vi "Actor Core.vi"(8 "error in":errorcluster, 11 "CS++DSCMonitor in":refnum<class "CS++DSCMonitor.lvclass">) -> (0 "error out":errorcluster, 3 "Actor out":refnum<class "Actor.lvclass">)   [LabVIEW 2014, in "CS++DSCMonitor.lvlib" / "CS++DSCMonitor.lvclass"]
doc: "(<B>Filename</B>: Actor Framework.lvlib:Actor.lvclass:Actor Core.vi)\n\nReceives messages to the actor, reacts to them, and initiates any error handling that may shut the actor down.\n\nDescendant classes may override this VI to append parallel tasks for the actor to complete while it handles messages. Overrides use the Call Parent Method node."
uses:
  CS++DSCMonitor.lvclass
  CSPP_Core/Actors/CS++SVMonitor/CS++SVMonitor.lvclass
  CSPP_Core/Actors/CS++BaseActor/CS++BaseActor.lvclass
  <vilib>/lvdsc/NI_DSC.lvlib
  <vilib>/ActorFramework/Actor/Actor.lvclass
  CSPP_Core/Actors/CS++PVMonitor Messages/CS++PVUpdate Msg/CS++PVUpdate Msg.lvclass
  CSPP_Core/Actors/CS++PVMonitor Messages/CS++AEUpdate Msg/CS++AEUpdate Msg.lvclass
  CSPP_Core/Classes/CS++ProcessVariables/AlarmEvent/AE.lvclass
  CSPP_Core/Classes/CS++ProcessVariables/AE Type.ctl
  CSPP_Core/Classes/CS++ProcessVariables/CS++ProcessVariables.lvlib
  CSPP_Core/Classes/CS++ProcessVariables/ProcessVariable/PV.lvclass
  <vilib>/ActorFramework/Report Error Msg/Report Error Msg.lvclass
  <vilib>/ActorFramework/Message Enqueuer/Message Priority.ctl
  <vilib>/ActorFramework/Message Enqueuer/Message Enqueuer.lvclass
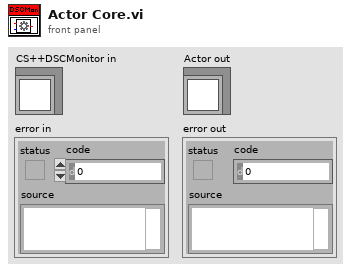
[diagram p1: front panel]
types:
  T1 = typedef "Actor Framework.lvlib/Message Enqueuer.lvclass/Message Priority.ctl" = enum16{"Low", "Normal", "High"}
  T2 = typedef "CS++ProcessVariables.lvlib/AE Type.ctl" = enum16{"Event", "HI_HI", "HI", "LO", "LO_LO", "Boolean", "ROC", "Invalid", "Other"}
  T3 = cluster{"Stop":refnum<user-event>, "PV Connections":refnum<user-event>}
  T4 = cluster{"PV URL":string, "Observers":cluster{"Enqueuer":refnum<class "Message Enqueuer.lvclass">, "CS++PVUpdate Msg":refnum<class "CS++PVUpdate Msg.lvclass">}[]}[]
  T5 = cluster{"AE URL":string, "Observers":cluster{"Enqueuer":refnum<class "Message Enqueuer.lvclass">, "CS++AEUpdate Msg":refnum<class "CS++AEUpdate Msg.lvclass">}[]}[]
  T6 = cluster{"PV URL":string, "Observers":cluster{"Enqueuer":refnum<class "Message Enqueuer.lvclass">, "CS++PVUpdate Msg":refnum<class "CS++PVUpdate Msg.lvclass">}[]}
  T7 = cluster{"Enqueuer":refnum<class "Message Enqueuer.lvclass">, "CS++PVUpdate Msg":refnum<class "CS++PVUpdate Msg.lvclass">}[]
  T8 = cluster{"AE URL":string, "Observers":cluster{"Enqueuer":refnum<class "Message Enqueuer.lvclass">, "CS++AEUpdate Msg":refnum<class "CS++AEUpdate Msg.lvclass">}[]}
  T9 = cluster{"Enqueuer":refnum<class "Message Enqueuer.lvclass">, "CS++AEUpdate Msg":refnum<class "CS++AEUpdate Msg.lvclass">}[]
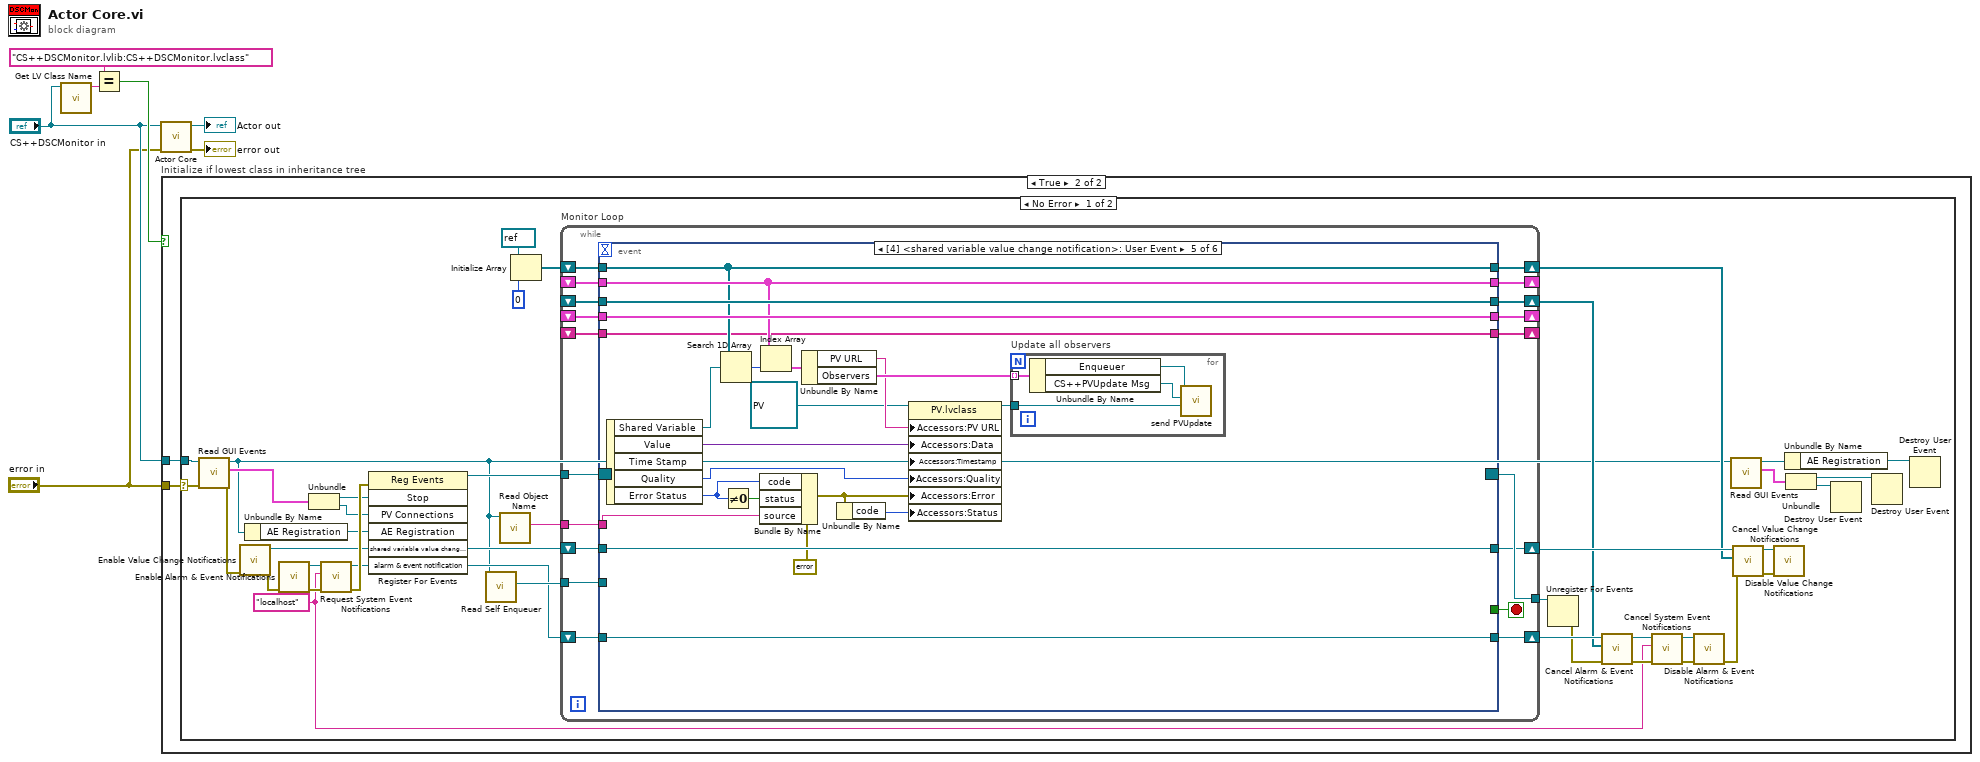
[diagram p0: block diagram]
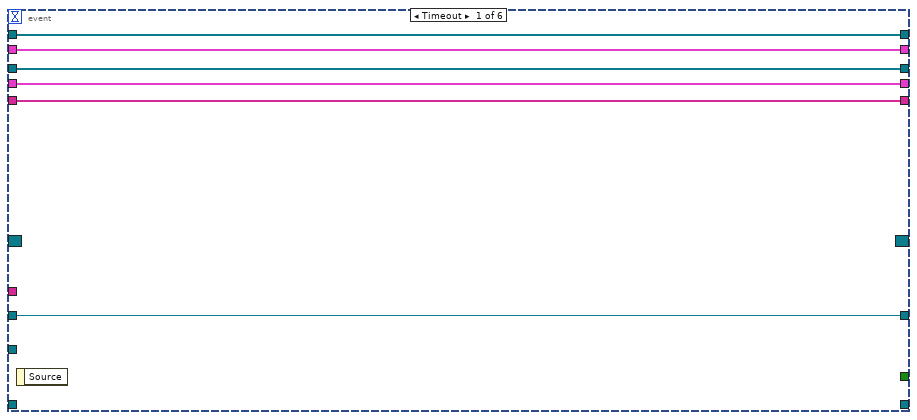
[diagram p3: hidden frame]
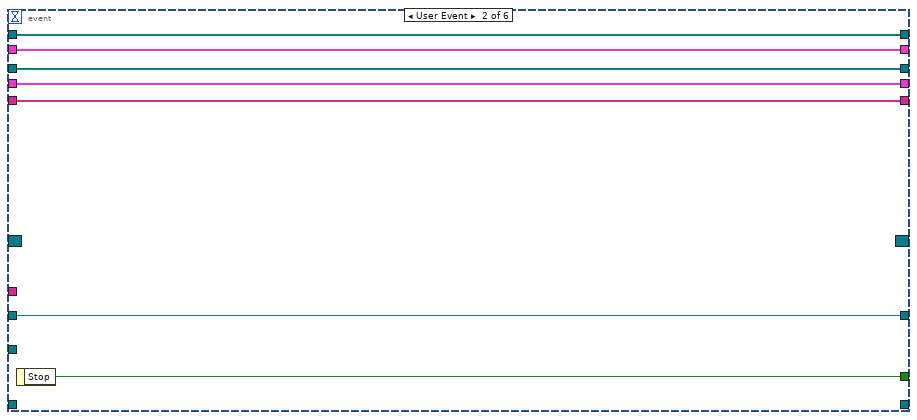
[diagram p4: hidden frame]
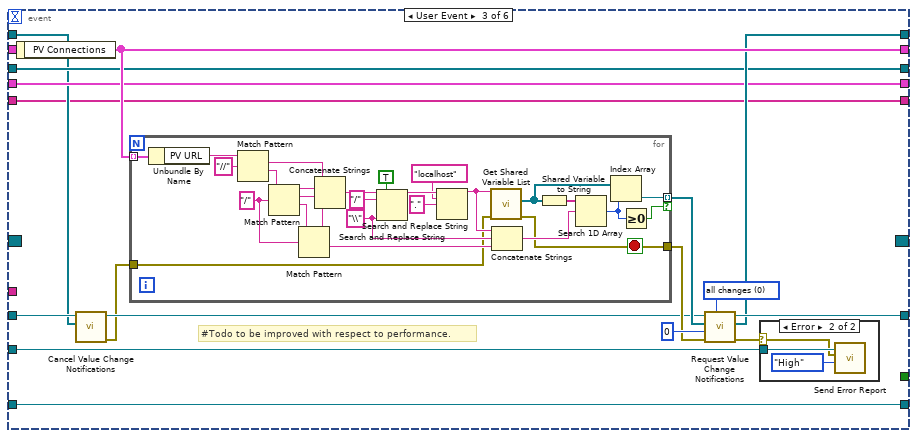
[diagram p5: hidden frame]
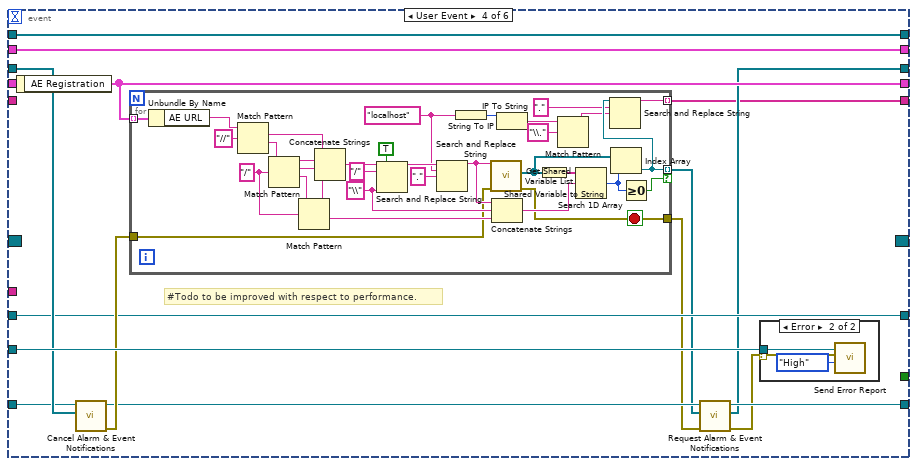
[diagram p7: hidden frame]
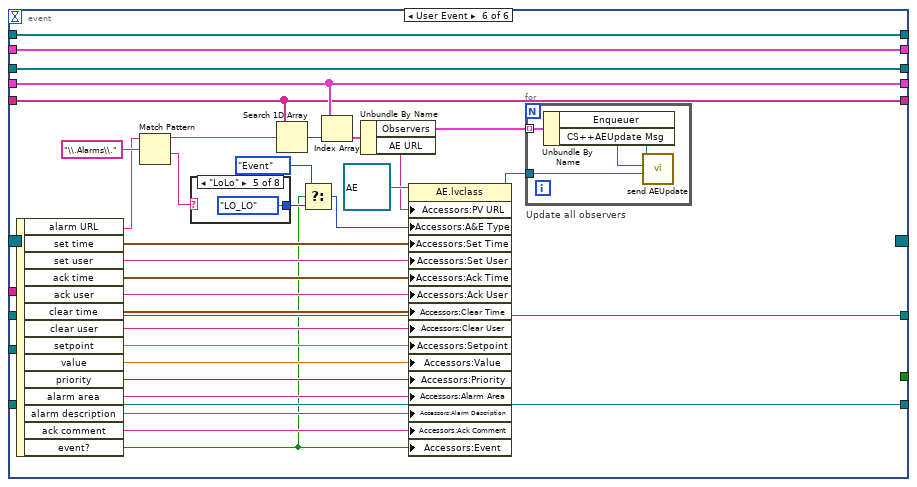
[diagram p9: hidden frame]
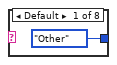
[diagram p10: hidden frame]
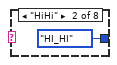
[diagram p11: hidden frame]
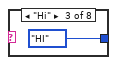
[diagram p12: hidden frame]
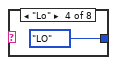
[diagram p13: hidden frame]
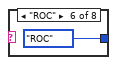
[diagram p14: hidden frame]
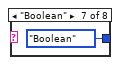
[diagram p15: hidden frame]
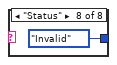
[diagram p16: hidden frame]
diagram:
  n1 = call <vilib>:"Get LV Class Name.vi"("object"="CS++DSCMonitor in") -> ("class name"=w6:string)  [unwired: 9 in, 1 out]
  n2 = Equal?(x="CS++DSCMonitor.lvlib:CS++DSCMonitor.lvclass" ("class name"), y=w6) -> (x = y?=w3:bool)
  n3 = call-parent "Actor Core.vi"("error in"="error in", "CS++SVMonitor in"="CS++DSCMonitor in") -> ("error out"=→"error out":errorcluster, "Actor out"=→"Actor out":refnum<class "Actor.lvclass">)  [unwired: 8 in]
  n4 = case "Initialize if lowest class in inheritance tree" shown="True" w3 {
    tunnel: "error in" -> [_ w9]
    tunnel: "CS++DSCMonitor in" -> [_ w8]
    frame False {
    }
    frame True {
      n5 = case shown="No Error" w9 {
        selector: w9 -> [w20 _]
        tunnel: w8 -> [w19 _]
        frame No Error {
          w18 = "localhost" ("server (localhost)")
          n6 = call "Read GUI Events.vi"("error in (no error)"=w20, "CS++SVMonitor in"=w19) -> ("error out"=w25:errorcluster, "GUI Events"=w24:T3, "CS++SVMonitor out"=w13:refnum<class "CS++DSCMonitor.lvclass">)  [unwired: 7 in]
          n7 = call <vilib>:"Enable Value Change Notifications.vi"("error in (no error)"=w25) -> ("error out"=w26:errorcluster, "shared variable value change notification"=w17:refnum<user-event>)  [unwired: 9 out]
          n8 = Unbundle By Name(w13) -> ("AE Registration"=w27:refnum<user-event>)
          n9 = call <vilib>:"Enable Alarm & Event Notifications.vi"("error in (no error)"=w26) -> ("error out"=w29:errorcluster, "alarm & event notification"=w28:refnum<user-event>)  [unwired: 9 out]
          n10 = Unbundle(w24) -> ("Stop"=w23:refnum<user-event>, "PV Connections"=w22:refnum<user-event>)
          n11 = call <vilib>:"Request System Event Notifications.vi"("error in (no error)"=w29, "server (localhost)"=w18, "notification refnum"=w28) -> ("error out"=w30:errorcluster, "alarm & event notification"=w16:refnum<user-event>)  [unwired: 6 in, 1 out]
          n12 = register-events(error in=w30, w23, w22, w27, w17, w16) -> (reference out=w21:refnum<event-registration>)  [unwired: 1 in, 1 out]
          n13 = call <vilib>:"Read Self Enqueuer.vi"("Actor"=w13) -> ("Self Enqueuer"=w44:refnum<class "Message Enqueuer.lvclass">)  [unwired: 10 in]
          n14 = call "Read Object Name.vi"("CS++BaseActor in"=w13) -> ("Object Name"=w46:string)  [unwired: 8 in, 2 out]
          n15 = Initialize Array(refnum<k21> refnum ("Shared Variable"), 0 ("dimension size")) -> (w43:refnum<k21>[])
          n16 = while "Monitor Loop" {
            tunnel: w21 -> [w67]
            tunnel: [w65] -> w48
            shift-right: [w63] -> w40
            shift-left: w43 -> [w64]
            shift-right: [w62] -> _
            shift-left: _ -> [w61]
            shift-right: [w59] -> w42
            shift-left: w17 -> [w60]
            tunnel: w46 -> [w58]
            tunnel: w44 -> [w57]
            shift-right: [w56] -> w38
            shift-left: w16 -> [w55]
            shift-right: [w52] -> w35
            shift-left: _ -> [w54]
            shift-right: [w53] -> _
            shift-left: _ -> [w51]
            shift-right: [w50] -> _
            shift-left: _ -> [w49]
            stop <- w66 stop-if-true
            n17 = event shown="[4] <shared variable value change notification>: User Event" {
              selector: w67 -> [_ _ _ _ _ _]
              dyn-events: [_ _ _ _ _ _] -> w65
              timeout: _ -> [_ _ _ _ _ _]
              tunnel: [_ w80 _ _ _ _] -> w66
              tunnel: w64 -> [w73 w79 w82 w138 w193 w235]
              tunnel: [w73 w79 w89 w138 w193 w235] -> w63
              tunnel: [w72 w78 w96 w141 w194 w237] -> w62
              tunnel: w61 -> [w72 w78 _ w141 w194 w237]
              tunnel: w60 -> [w71 w77 w85 w135 w201 w238]
              tunnel: [w71 w77 w97 w135 w201 w238] -> w59
              tunnel: w58 -> [_ _ _ _ w191 _]
              tunnel: w57 -> [_ _ w91 w142 _ _]
              tunnel: [_ _ w90 w133 w197 w236] -> w56
              tunnel: w55 -> [_ _ w90 w136 w197 w236]
              tunnel: w54 -> [w69 w76 w87 w139 w196 w234]
              tunnel: [w70 w75 w86 w140 w195 w233] -> w53
              tunnel: [w69 w76 w87 w130 w196 w234] -> w52
              tunnel: w51 -> [w70 w75 w86 _ w195 w233]
              tunnel: [w68 w74 w81 w128 w188 w229] -> w50
              tunnel: w49 -> [w68 w74 w81 _ w188 w229]
              event Timeout {
                n18 = event-data() -> ()  [unwired: 1 in, 1 out]
              }
              event User Event {
                n19 = event-data() -> ("Stop"=w80:bool)  [unwired: 1 in]
              }
              event User Event {
                w95 = u16 0 items=["all changes", "value changes only"] ("request changes (all changes)")
                # "#Todo to be improved with respect to performance."
                n20 = event-data() -> ("PV Connections"=w96:T4)  [unwired: 1 in]
                n21 = call <vilib>:"Cancel Value Change Notifications.vi"("shared variables"=w82, "notification refnum"=w85) -> ("error out"=w83:errorcluster, "shared variable value change notification"=w84:refnum<user-event>)  [unwired: 1 in, 7 out]
                n22 = for {
                  tunnel: w96 -> [w127] mode=indexing
                  tunnel: [w115] -> w88 mode=indexing if=w114
                  tunnel: [w102] -> w93
                  tunnel: w83 -> [w101]
                  stop <- w102 stop-if-true
                  w103 = "\\" ("replace string (\"\")")
                  w123 = "/" ("regular expression")
                  n23 = Unbundle By Name(w127) -> ("PV URL"=w117:string)
                  n24 = Match Pattern(string=w117, regular expression="//") -> (match substring=w122:string, after substring=w125:string)  [unwired: 1 in, 2 out]
                  n25 = Match Pattern(string=w125, regular expression=w123) -> (before substring=w121:string, match substring=w120:string, after substring=w124:string)  [unwired: 1 in, 1 out]
                  n26 = Match Pattern(string=w124, regular expression=w123) -> (before substring=w119:string, after substring=w109:string)  [unwired: 1 in, 2 out]
                  n27 = Concatenate Strings(w122, w121, w120, w119) -> (w112:string)
                  n28 = Search and Replace String(replace all?=TRUE ("replace all? (F)"), input string=w112, search string="/", replace string=w103) -> (result string=w107:string)  [unwired: 4 in, 3 out]
                  n29 = Search and Replace String(input string=w107, search string="localhost", replace string="." ("replace string (\"\")")) -> (result string=w104:string)  [unwired: 5 in, 3 out]
                  n30 = call <vilib>:"Get Shared Variable List.vi"("error in (no error)"=w101, "process name"=w104) -> ("error out"=w102:errorcluster, "shared variables"=w116:refnum<k21>[])  [unwired: 8 out]
                  n31 = Concatenate Strings(w104, w103, w109) -> (w108:string)
                  n32 = Shared Variable to String(1:w116) -> (0:w118:string[])
                  n33 = Search 1D Array(1D array=w118, element=w108) -> (index of element=w113:i32)  [unwired: 1 in]
                  n34 = Index Array(array=w116, index=w113) -> (element=w115:refnum<k21>)
                  n35 = Greater Or Equal To 0?(x=w113) -> (x >= 0?=w114:bool)
                }
                n36 = call <vilib>:"Request Value Change Notifications.vi"("request changes (all changes)"=w95, "error in (no error)"=w93, "updates to buffer (no buffer)"=u32 0, "shared variables"=w88, "notification refnum"=w84) -> ("error out"=w92:errorcluster, "shared variables out"=w89:refnum<k21>[], "shared variable value change notification"=w97:refnum<user-event>)  [unwired: 4 out]
                n37 = case shown="Error" w92 {
                  selector: w92 -> [_ w99]
                  tunnel: w91 -> [_ w100]
                  frame No Error {
                  }
                  frame Error {
                    n38 = call <vilib>:"Send Error Report.vi"("Message Priority (Normal)"=Message_Priority."High", "Error From Sender"=w99, "Message Enqueuer"=w100) -> ()  [unwired: 8 in, 1 out]
                  }
                }
              }
              event User Event {
                # "#Todo to be improved with respect to performance."
                n39 = event-data() -> ("AE Registration"=w140:T5)  [unwired: 1 in]
                n40 = call <vilib>:"Cancel Alarm & Event Notifications.vi"("shared variables"=w139, "notification refnum"=w136) -> ("error out"=w137:errorcluster, "alarm & event notification"=w134:refnum<user-event>)  [unwired: 7 in, 1 out]
                n41 = for {
                  tunnel: w140 -> [w178] mode=indexing
                  tunnel: [w150] -> w129 mode=indexing if=w167
                  tunnel: [w157] -> w132
                  tunnel: w137 -> [w156]
                  tunnel: [w151] -> w128 mode=indexing
                  stop <- w157 stop-if-true
                  w153 = "localhost" ("search string")
                  w158 = "\\" ("replace string (\"\")")
                  w174 = "/" ("regular expression")
                  n42 = Unbundle By Name(w178) -> ("AE URL"=w152:string)
                  n43 = Match Pattern(string=w152, regular expression="//") -> (match substring=w173:string, after substring=w176:string)  [unwired: 1 in, 2 out]
                  n44 = Match Pattern(string=w176, regular expression=w174) -> (before substring=w172:string, match substring=w171:string, after substring=w175:string)  [unwired: 1 in, 1 out]
                  n45 = Match Pattern(string=w175, regular expression=w174) -> (before substring=w170:string, after substring=w162:string)  [unwired: 1 in, 2 out]
                  n46 = Concatenate Strings(w173, w172, w171, w170) -> (w165:string)
                  n47 = Search and Replace String(replace all?=TRUE ("replace all? (F)"), input string=w165, search string="/", replace string=w158) -> (result string=w160:string)  [unwired: 4 in, 3 out]
                  n48 = Search and Replace String(input string=w160, search string=w153, replace string="." ("replace string (\"\")")) -> (result string=w159:string)  [unwired: 5 in, 3 out]
                  n49 = String To IP(1:w153) -> (0:w155:u32)
                  n50 = call <vilib>:"Get Shared Variable List.vi"("error in (no error)"=w156, "process name"=w159) -> ("error out"=w157:errorcluster, "shared variables"=w168:refnum<k21>[])  [unwired: 8 out]
                  n51 = Concatenate Strings(w159, w158, w162) -> (w161:string)
                  n52 = IP To String(2:w155) -> (0:w154:string)  [unwired: 1 in]
                  n53 = Shared Variable to String(1:w168) -> (0:w169:string[])
                  n54 = Match Pattern(string=w154, regular expression="\\.") -> (before substring=w149:string)  [unwired: 1 in, 3 out]
                  n55 = Search 1D Array(1D array=w169, element=w161) -> (index of element=w166:i32)  [unwired: 1 in]
                  n56 = Index Array(array=w168, index=w166) -> (element=w150:refnum<k21>)
                  n57 = Search and Replace String(input string=w150, search string=".", replace string=w149) -> (result string=w151:string)  [unwired: 5 in, 3 out]
                  n58 = Greater Or Equal To 0?(x=w166) -> (x >= 0?=w167:bool)
                }
                n59 = call <vilib>:"Request Alarm & Event Notifications.vi"("error in (no error)"=w132, "shared variables"=w129, "notification refnum"=w134) -> ("error out"=w131:errorcluster, "shared variables out"=w130:refnum<k21>[], "alarm & event notification"=w133:refnum<user-event>)  [unwired: 6 out]
                n60 = case shown="Error" w131 {
                  selector: w131 -> [_ w144]
                  tunnel: w142 -> [_ w145]
                  frame No Error {
                  }
                  frame Error {
                    n61 = call <vilib>:"Send Error Report.vi"("Message Priority (Normal)"=Message_Priority."High", "Error From Sender"=w144, "Message Enqueuer"=w145) -> ()  [unwired: 8 in, 1 out]
                  }
                }
              }
              event User Event {
                n62 = event-data() -> ("Shared Variable"=w198:refnum<k21>, "Value"=w184:variant, "Time Stamp"=w183:timestamp, "Quality"=w181:u64, "Error Status"=w189:i32)  [unwired: 1 in]
                n63 = Search 1D Array(1D array=w193, element=w198) -> (index of element=w200:i32)  [unwired: 1 in]
                n64 = Not Equal To 0?(x=w189) -> (x != 0?=w190:bool)
                n65 = Bundle By Name(cluster=errorcluster {"status"=FALSE, "code"=0, "source"=""} ("Error"), "code"=w189, "status"=w190, "source"=w191) -> (w182:errorcluster)
                n66 = Index Array(array=w194, index=w200) -> (element=w199:T6)
                n67 = Unbundle By Name(w199) -> ("PV URL"=w185:string, "Observers"=w187:T7)
                n68 = Unbundle By Name(w182) -> ("code"=w186:i32)
                n69 = property class="PV.lvclass"(reference=refnum<class "PV.lvclass"> refnum ("PV"), "Accessors:PV URL"=w185, "Accessors:Data"=w184, "Accessors:Timestamp"=w183, "Accessors:Quality"=w181, "Accessors:Error"=w182, "Accessors:Status"=w186) -> (reference out=w180:refnum<class "PV.lvclass">)  [unwired: 1 in, 1 out]
                n70 = for "Update all observers" {
                  tunnel: w187 -> [w205] mode=indexing
                  tunnel: w180 -> [w202]
                  n71 = Unbundle By Name(w205) -> ("Enqueuer"=w204:refnum<class "Message Enqueuer.lvclass">, "CS++PVUpdate Msg"=w203:refnum<class "CS++PVUpdate Msg.lvclass">)
                  n72 = call "send PVUpdate.vi"("PV"=w202, "CS++PVUpdate Msg in"=w203, "Message Enqueuer in"=w204) -> ()  [unwired: 7 in, 2 out]
                }
              }
              event User Event {
                n73 = event-data() -> ("alarm URL"=w227:string, "set time"=w219:timestamp, "set user"=w218:string, "ack time"=w217:timestamp, "ack user"=w216:string, "clear time"=w215:timestamp, "clear user"=w214:string, "setpoint"=w213:dbl, "value"=w212:dbl, "priority"=w211:u32, "alarm area"=w210:string, "alarm description"=w209:string, "ack comment"=w208:string, "event?"=w207:bool)  [unwired: 1 in]
                n74 = Match Pattern(string=w227, regular expression="\\.Alarms\\.") -> (before substring=w225:string, after substring=w224:string)  [unwired: 1 in, 2 out]
                n75 = case shown="\"LoLo\"" w224 {
                  tunnel: [AE_Type."Other" ("A&E Type") AE_Type."HI_HI" ("A&E Type") AE_Type."HI" ("A&E Type") AE_Type."LO" ("A&E Type") AE_Type."LO_LO" ("A&E Type") AE_Type."ROC" ("A&E Type") AE_Type."Boolean" ("A&E Type") AE_Type."Invalid" ("A&E Type")] -> w221
                  frame Default {
                  }
                  frame "HiHi" {
                  }
                  frame "Hi" {
                  }
                  frame "Lo" {
                  }
                  frame "LoLo" {
                  }
                  frame "ROC" {
                  }
                  frame "Boolean" {
                  }
                  frame "Status" {
                  }
                }
                n76 = Search 1D Array(1D array=w229, element=w225) -> (index of element=w231:i32)  [unwired: 1 in]
                n77 = Select(t=AE_Type."Event" ("A&E Type"), s=w207, f=w221) -> (s? t:f=w222:T2)
                n78 = Index Array(array=w233, index=w231) -> (element=w230:T8)
                n79 = Unbundle By Name(w230) -> ("Observers"=w232:T9, "AE URL"=w220:string)
                n80 = property class="AE.lvclass"(reference=refnum<class "AE.lvclass"> refnum ("CS++ProcessVariables.lvlib:AE.lvclass"), "Accessors:PV URL"=w220, "Accessors:A&E Type"=w222, "Accessors:Set Time"=w219, "Accessors:Set User"=w218, "Accessors:Ack Time"=w217, "Accessors:Ack User"=w216, "Accessors:Clear Time"=w215, "Accessors:Clear User"=w214, "Accessors:Setpoint"=w213, "Accessors:Value"=w212, "Accessors:Priority"=w211, "Accessors:Alarm Area"=w210, "Accessors:Alarm Description"=w209, "Accessors:Ack Comment"=w208, "Accessors:Event"=w207) -> (reference out=w206:refnum<class "AE.lvclass">)  [unwired: 1 in, 1 out]
                n81 = for "Update all observers" {
                  tunnel: w232 -> [w250] mode=indexing
                  tunnel: w206 -> [w247]
                  n82 = Unbundle By Name(w250) -> ("Enqueuer"=w249:refnum<class "Message Enqueuer.lvclass">, "CS++AEUpdate Msg"=w248:refnum<class "CS++AEUpdate Msg.lvclass">)
                  n83 = call "send AEUpdate.vi"("AE"=w247, "CS++AEUpdate Msg in"=w248, "Message Enqueuer in"=w249) -> ()  [unwired: 7 in, 2 out]
                }
              }
            }
          }
          n84 = Unregister For Events(event registration refnum=w48) -> (error out=w36:errorcluster)  [unwired: 1 in]
          n85 = call <vilib>:"Cancel Alarm & Event Notifications.vi"("error in (no error)"=w36, "shared variables"=w35, "notification refnum"=w38) -> ("error out"=w32:errorcluster, "alarm & event notification"=w34:refnum<user-event>)  [unwired: 6 in, 1 out]
          n86 = call <vilib>:"Cancel System Event Notifications.vi"("error in (no error)"=w32, "server (localhost)"=w18, "notification refnum"=w34) -> ("error out"=w31:errorcluster, "alarm & event notification"=w33:refnum<user-event>)  [unwired: 6 in, 1 out]
          n87 = call <vilib>:"Disable Alarm & Event Notifications.vi"("error in (no error)"=w31, "notification refnum"=w33) -> ("error out"=w37:errorcluster)  [unwired: 9 out]
          n88 = call "Read GUI Events.vi"("CS++SVMonitor in"=w13) -> ("GUI Events"=w14:T3, "CS++SVMonitor out"=w15:refnum<class "CS++DSCMonitor.lvclass">)  [unwired: 8 in, 1 out]
          n89 = call <vilib>:"Cancel Value Change Notifications.vi"("error in (no error)"=w37, "shared variables"=w40, "notification refnum"=w42) -> ("error out"=w39:errorcluster, "shared variable value change notification"=w41:refnum<user-event>)  [unwired: 7 out]
          n90 = call <vilib>:"Disable Value Change Notifications.vi"("error in (no error)"=w39, "notification refnum"=w41) -> ()  [unwired: 10 out]
          n91 = Unbundle By Name(w15) -> ("AE Registration"=w12:refnum<user-event>)
          n92 = Unbundle(w14) -> ("Stop"=w10:refnum<user-event>, "PV Connections"=w11:refnum<user-event>)
          n93 = Destroy User Event(user event=w11) -> ()  [unwired: 1 in, 1 out]
          n94 = Destroy User Event(user event=w10) -> ()  [unwired: 1 in, 1 out]
          n95 = Destroy User Event(user event=w12) -> ()  [unwired: 1 in, 1 out]
        }
        frame Error {
        }
      }
    }
  }
